vi "Set separate code.vi"() -> ()   [LabVIEW 2016]
panel:
  in  "Open bad":bool=TRUE
  in  "Stop on bad":bool=TRUE
  out "Execution:State":T1(ring)
  out "Modified files":path[](array[path])
  out "Modified":i32
  in  "Stop Button":bool
  out "File Path":path
  out "Progress":string
  in  "Folder Path":path
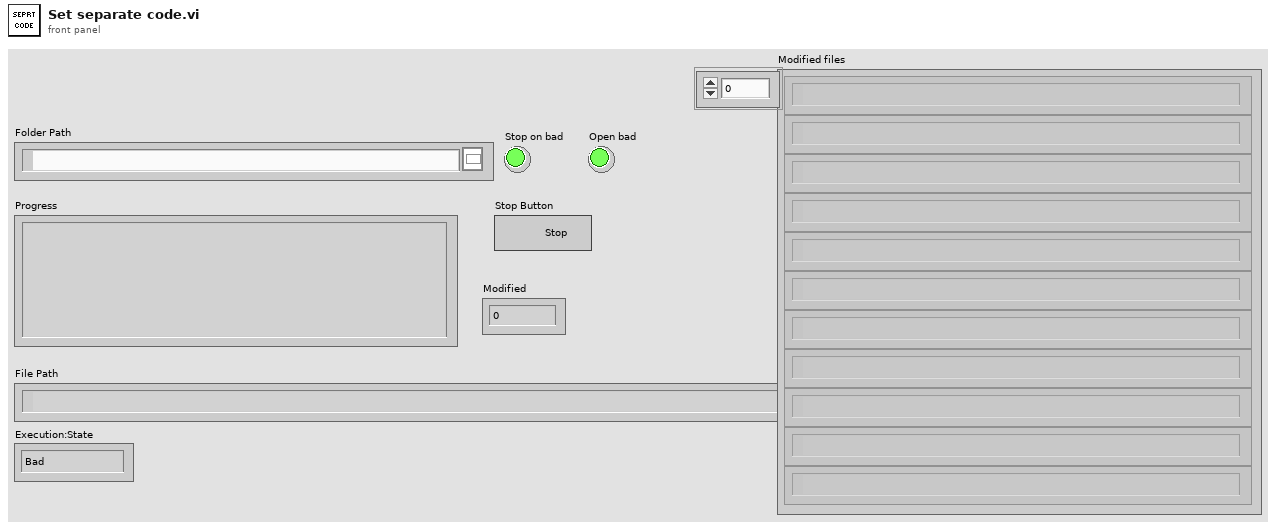
[diagram p1: front panel]
types:
  T1 = enum32{"Bad", "Idle", "Run top level", "Running"}
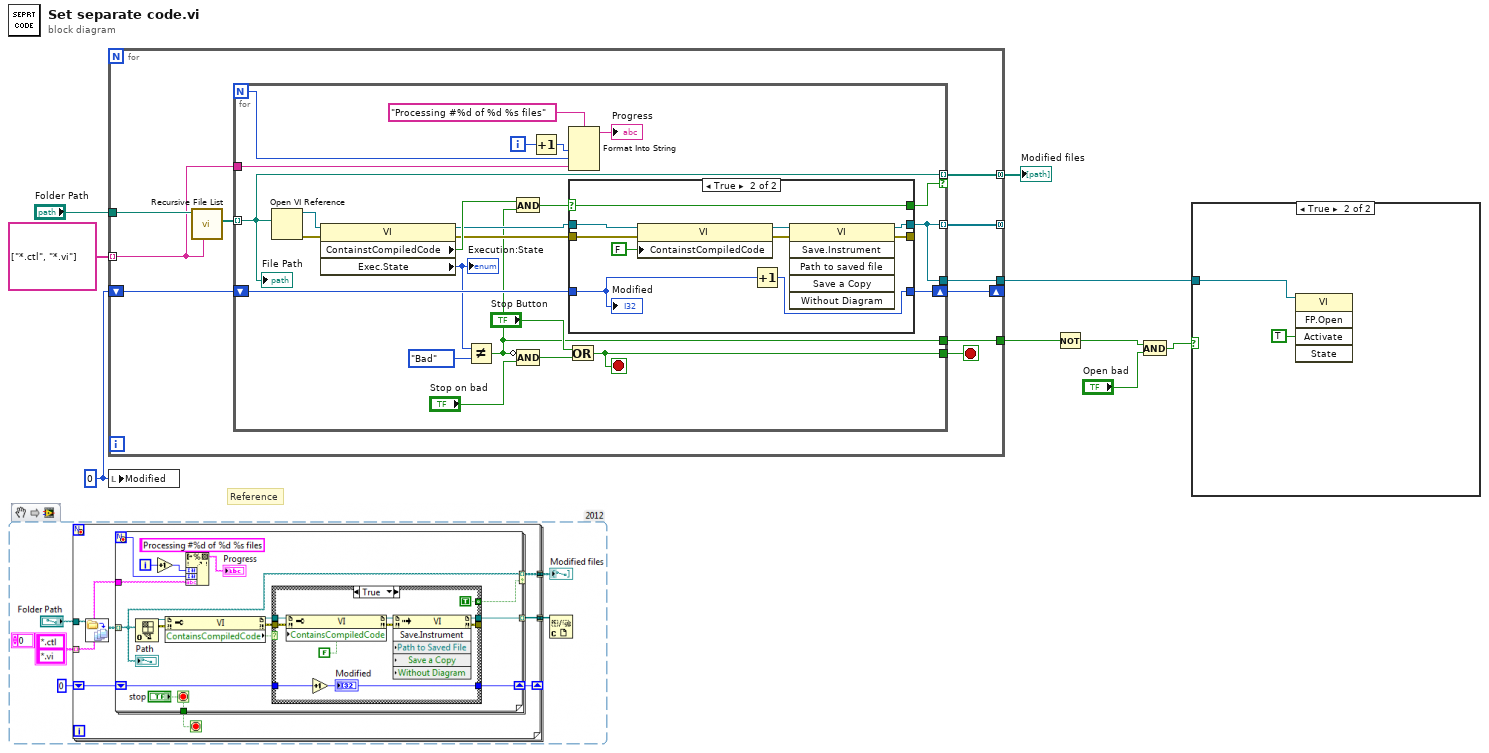
[diagram p0: block diagram]
diagram:
  w6 = 0 ("Modified")
  # "Reference"
  n1 = for {
    tunnel: string[] ["*.ctl", "*.vi"] -> [w17] mode=indexing
    shift-right: [w14] -> _
    shift-left: w6 -> [w15]
    tunnel: "Folder Path" -> [w19]
    tunnel: [w13] -> _ mode=concatenating
    tunnel: [w12] -> w7 mode=concatenating
    tunnel: [w11] -> w5
    tunnel: [w10] -> w3
    stop <- w16 stop-if-true
    n2 = call <vilib>:"Recursive File List.vi"("pattern"=w17, "Folder Path"=w19) -> ("All Files in Dir"=w18:path[])  [unwired: 5 in, 4 out]
    n3 = for {
      N -> [w40]
      tunnel: w18 -> [w29] mode=indexing
      tunnel: w17 -> [w39]
      tunnel: [w23] -> w16
      tunnel: [w21] -> w13 mode=indexing
      shift-right: [w30] -> w14
      shift-left: w15 -> [w31]
      tunnel: [w29] -> w12 mode=indexing if=w28
      tunnel: [w21] -> w11
      tunnel: [w20] -> w10
      i -> [w42]
      stop <- w23 stop-if-true
      n4 = Open VI Reference(vi path=w29) -> (vi reference=w37:refnum<vi>, error out=w36:errorcluster)  [unwired: 5 in]
      n5 = property class="VI"(reference=w37, error in=w36) -> (reference out=w33:refnum<vi>, error out=w32:errorcluster, "ContainstCompiledCode"=w34:bool, "Exec.State"=w27:T1)
      "Execution:State" <- w27
      n6 = Not Equal?(x=w27, y=T1."Bad" ("Execution:State")) -> (x != y?=w20:bool)
      n7 = And(x=w34, y=w20) -> (x .and. y?=w25:bool)
      n8 = Compound Arithmetic op=AND(invert w20, "Stop on bad") -> (w22:bool)
      n9 = Increment(x=w42) -> (x+1=w41:i32)
      n10 = Or(x="Stop Button", y=w22) -> (x .or. y?=w23:bool)
      n11 = Format Into String(format string="Processing #%d of %d %s files", w41, w40, w39) -> (resulting string=→"Progress":string)  [unwired: 2 in, 1 out]
      n12 = case shown="True" w25 {
        selector: w25 -> [w44 w49]
        tunnel: w33 -> [w46 w56]
        tunnel: w32 -> [w47 w55]
        tunnel: [w47 w52] -> _
        tunnel: [w46 w51] -> w21
        tunnel: w31 -> [w45 w48]
        tunnel: [w45 w50] -> w30
        tunnel: [w44 w49] -> w28
        frame False {
        }
        frame True {
          n13 = property class="VI"(reference=w56, error in=w55, "ContainstCompiledCode"=FALSE ("Contains Compiled Code")) -> (reference out=w54:refnum<vi>, error out=w53:errorcluster)
          n14 = Increment(x=w48) -> (x+1=w50:i32)
          n15 = invoke class="VI" method="Save.Instrument"(reference=w54, error in=w53) -> (reference out=w51:refnum<vi>, error out=w52:errorcluster)  [unwired: 4 in, 4 out]
          "Modified" <- w48
        }
      }
      "File Path" <- w29
    }
  }
  "Modified files" <- w7
  n16 = local write "Modified"(w6) -> ()
  n17 = Not(x=w3) -> (.not. x?=w1:bool)
  n18 = And(x=w1, y="Open bad") -> (x .and. y?=w4:bool)
  n19 = case shown="True" w4 {
    tunnel: w5 -> [_ w59]
    frame False {
    }
    frame True {
      n20 = invoke class="VI" method="FP.Open"(reference=w59, "Activate"=TRUE ("Activate?")) -> ()  [unwired: 3 in, 5 out]
    }
  }
